vi "CloseAllComPorts.vi"() -> ()   [LabVIEW 2013]
panel:
  out "Array 2":refnum<visa-resource-name>[](array[refnum])
  out "Array":errorcluster[](array[cluster])
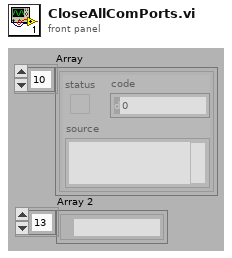
[diagram p1: front panel]
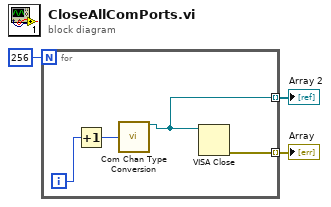
[diagram p0: block diagram]
diagram:
  n1 = for {
    N: 256 -> [_]
    tunnel: [w5] -> w2 mode=indexing
    tunnel: [w4] -> w1 mode=indexing
    i -> [w7]
    n2 = Increment(x=w7) -> (x+1=w6:i32)
    n3 = call "Com Chan Type Conversion.vi"("Com Chan"=w6) -> ("VISA resource name"=w4:refnum<visa-resource-name>)  [unwired: 11 in, 3 out]
    n4 = VISA Close(VISA resource name=w4) -> (error out=w5:errorcluster)  [unwired: 1 in]
  }
  "Array" <- w2
  "Array 2" <- w1
